vi "GetFormationTiming.vi"(10 "Hold off Guess":dbl, 11 "Trigger Data":T3) -> (3 "Formation Timing":dbl)   [LabVIEW 2016]
uses:
  Ctrl_Signal.ctl
  Ctrl_Signal_Map.ctl
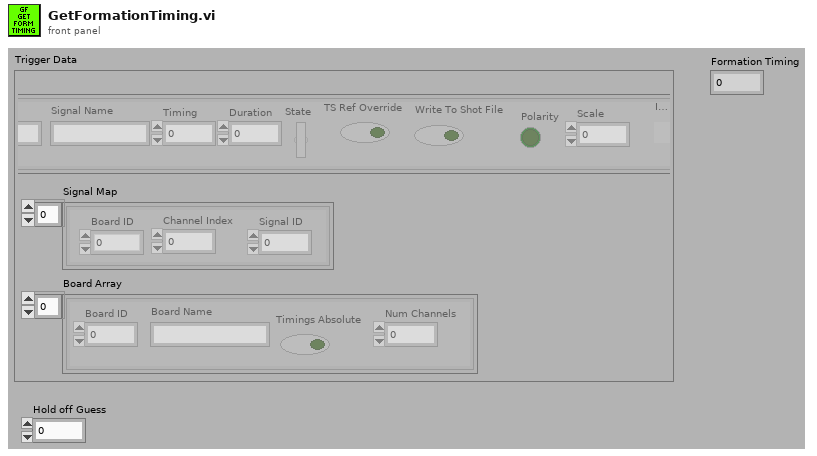
[diagram p1: front panel]
types:
  T1 = typedef "Ctrl_Signal.ctl" = cluster{"Signal Name":string, "Timing":dbl, "Duration":dbl, "State":bool, "TS Ref Override":bool, "Write To Shot File":bool, "Polarity":bool, "Signal ID":dbl, "Scale":dbl, "IsDelay":bool}
  T2 = typedef "Ctrl_Signal_Map.ctl" = cluster{"Channel Index":dbl, "Board ID":dbl, "Signal ID":dbl}
  T3 = cluster{"Signal Array":T1[], "Signal Map":T2[], "Board Array":cluster{"Board ID":dbl, "Board Name":string, "Timings Absolute":bool, "Num Channels":dbl}[]}
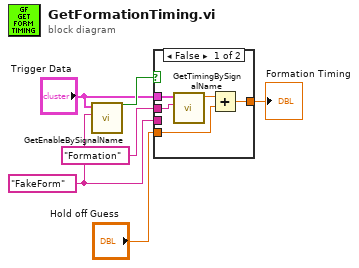
[diagram p0: block diagram]
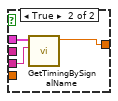
[diagram p2: hidden frame]
diagram:
  w5 = "FakeForm" ("Signal Name")
  n1 = call "GetEnableBySignalName.vi"("Signal Name"=w5, "Trigger Data"="Trigger Data") -> ("Signal Enabled"=w6:bool)  [unwired: 9 in]
  n2 = case shown="False" w6 {
    tunnel: "Trigger Data" -> [w11 w14]
    tunnel: w5 -> [_ w13]
    tunnel: "Formation" ("Signal Name") -> [w10 _]
    tunnel: "Hold off Guess" -> [w8 _]
    tunnel: [w7 w12] -> w1
    frame False {
      n3 = call "GetTimingBySignalName.vi"("Signal Name"=w10, "Trigger Data"=w11) -> ("Timing"=w9:dbl)  [unwired: 9 in]
      n4 = Add(x=w9, y=w8) -> (x+y=w7:dbl)
    }
    frame True {
      n5 = call "GetTimingBySignalName.vi"("Signal Name"=w13, "Trigger Data"=w14) -> ("Timing"=w12:dbl)  [unwired: 9 in]
    }
  }
  "Formation Timing" <- w1
